vi "Read UIRef.vi"(8 "error in (no error)":errorcluster, 9 "0Arrive/1Finish":i32, 10 "UI Ref":T1, 11 "NG Pick in":refnum<class "NG Pick.lvclass">) -> (0 "error out":errorcluster, 2 "RefOut":refnum<vi>, 3 "NG Pick out":refnum<class "NG Pick.lvclass">)   [LabVIEW 2019, in "NG Pick.lvclass"]
uses:
  NG Pick.lvclass
  Ctrl/Auto Inspection Main UI Ref.ctl
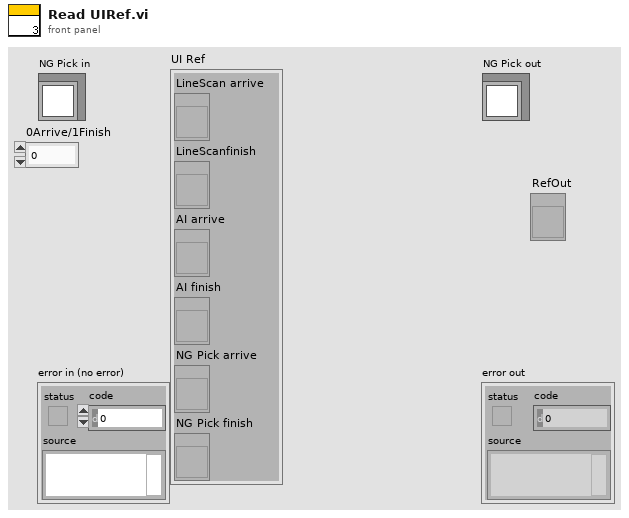
[diagram p1: front panel]
types:
  T1 = typedef "Auto Inspection Main UI Ref.ctl" = cluster{"LineScan arrive":refnum<vi>, "LineScanfinish":refnum<vi>, "AI arrive":refnum<vi>, "AI finish":refnum<vi>, "NG Pick arrive":refnum<vi>, "NG Pick finish":refnum<vi>}
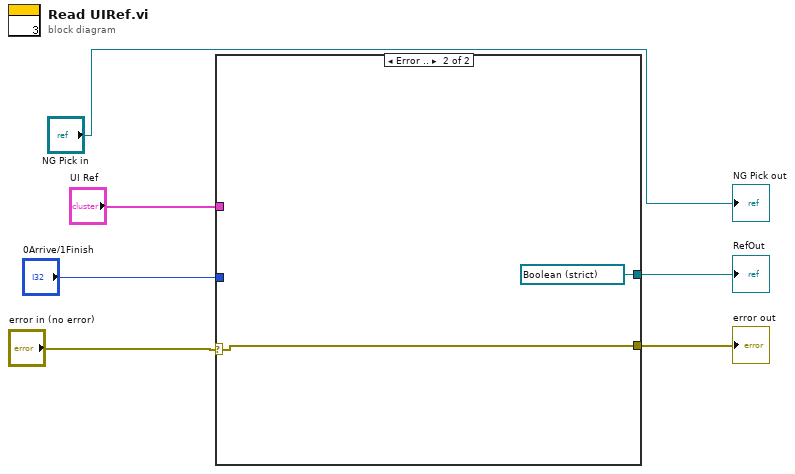
[diagram p0: block diagram]
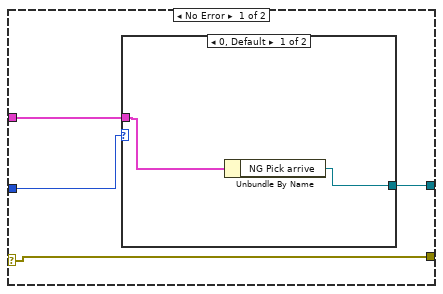
[diagram p2: hidden frame]
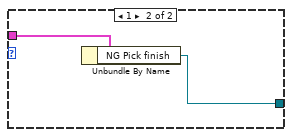
[diagram p3: hidden frame]
diagram:
  n1 = case shown="Error .." "error in (no error)" {
    selector: "error in (no error)" -> [w10 w15]
    tunnel: [w10 w15] -> w5
    tunnel: "UI Ref" -> [w8 _]
    tunnel: "0Arrive/1Finish" -> [w9 _]
    tunnel: [w7 refnum<vi> refnum ("NG Pick finish")] -> w1
    frame No Error {
      n2 = case shown="0, Default" w9 {
        tunnel: w8 -> [w12 w14]
        tunnel: [w11 w13] -> w7
        frame 0, Default {
          n3 = Unbundle By Name(w12) -> ("NG Pick arrive"=w11:refnum<vi>)
        }
        frame 1 {
          n4 = Unbundle By Name(w14) -> ("NG Pick finish"=w13:refnum<vi>)
        }
      }
    }
    frame Error {
    }
  }
  "error out" <- w5
  "RefOut" <- w1
  "NG Pick out" <- "NG Pick in"
